vi "Start.vi"(8 "error in (no error)":errorcluster, 11 "Motor-Maxon in":refnum<class "Motor-Maxon.lvclass">) -> (0 "error out":errorcluster, 3 "Motor-Maxon out":refnum<class "Motor-Maxon.lvclass">)   [LabVIEW 2013, in "PowderDeposition.lvlib" / "Motor-Maxon.lvclass"]
uses:
  Motor-Maxon.lvclass
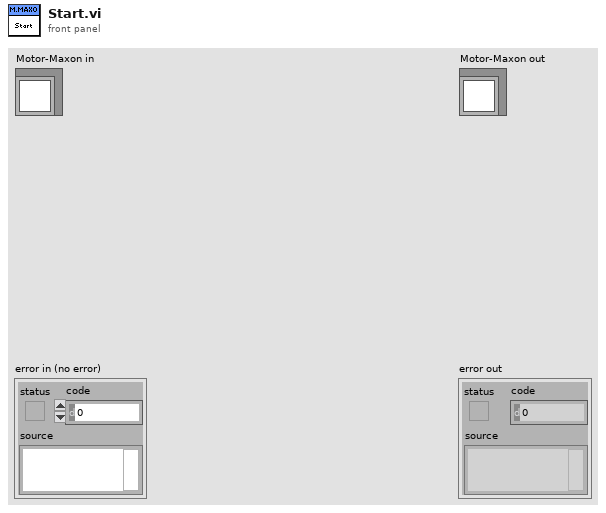
[diagram p1: front panel]
types:
  T1 = cluster{"profileAcceleration":u32, "profileDeceleration":u32}
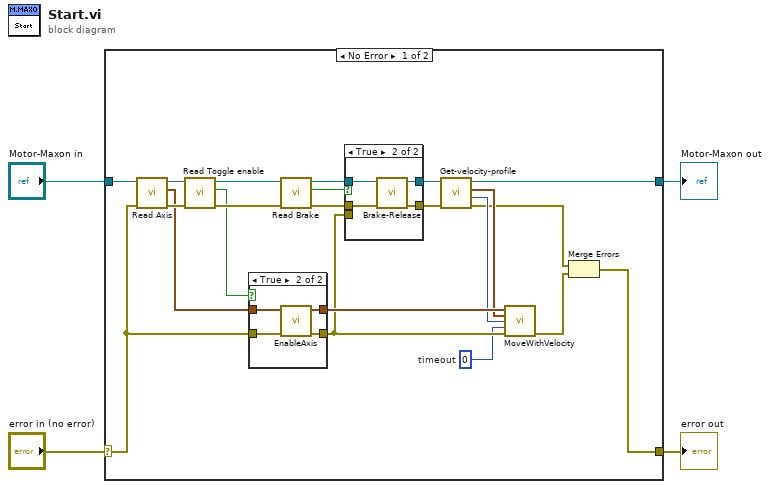
[diagram p0: block diagram]
diagram:
  n1 = case shown="No Error" "error in (no error)" {
    selector: "error in (no error)" -> [w9 w40]
    tunnel: [w26 w40] -> w3
    tunnel: [w7 w39] -> w1
    tunnel: "Motor-Maxon in" -> [w10 w39]
    frame No Error {
      w11 = u32 0  # timeout
      n2 = call-dynamic "Read Axis.vi"("error in (no error)"=w9, "Motor-Maxon in"=w10) -> ("error out"=w24:errorcluster, "Axis"=w23:cluster{"keyHandle":u32, "nodeID":u16}, "Motor-Maxon out"=w25:refnum<class "Motor-Maxon.lvclass">)  [unwired: 7 in]
      n3 = call-dynamic "Read Toggle enable.vi"("error in (no error)"=w24, "Motor-Maxon in"=w25) -> ("error out"=w21:errorcluster, "Toggle enable"=w12:bool, "Motor-Maxon out"=w22:refnum<class "Motor-Maxon.lvclass">)  [unwired: 7 in]
      n4 = case shown="True" w12 {
        tunnel: w23 -> [w34 w37]
        tunnel: w9 -> [w33 w38]
        tunnel: [w34 w36] -> w18
        tunnel: [w33 w35] -> w17
        frame False {
        }
        frame True {
          n5 = call <instrlib>:"EnableAxis.vi"("error in (no error)"=w38, "axis in"=w37) -> ("error out"=w35:errorcluster, "axis out"=w36:cluster{"keyHandle":u32, "nodeId":u16})  [unwired: 4 in]
        }
      }
      n6 = call-dynamic "Read Brake.vi"("error in (no error)"=w21, "Motor-Maxon in"=w22) -> ("error out"=w19:errorcluster, "Brake"=w13:bool, "Motor-Maxon out"=w20:refnum<class "Motor-Maxon.lvclass">)  [unwired: 7 in]
      n7 = case shown="True" w13 {
        tunnel: w20 -> [w28 w32]
        tunnel: w19 -> [w27 w31]
        tunnel: [w28 w30] -> w16
        tunnel: [w27 w29] -> w15
        tunnel: w17 -> [_ _]
        frame False {
        }
        frame True {
          n8 = call-dynamic "Brake-Release.vi"("error in (no error)"=w31, "Motor-Maxon in"=w32) -> ("error out"=w29:errorcluster, "Motor-Maxon out"=w30:refnum<class "Motor-Maxon.lvclass">)  [unwired: 8 in]
        }
      }
      n9 = call-dynamic "Get-velocity-profile.vi"("error in (no error)"=w15, "Motor-Maxon in"=w16) -> ("error out"=w6:errorcluster, "Velocity"=w8:i32, "Velocity profile"=w14:T1, "Motor-Maxon out"=w7:refnum<class "Motor-Maxon.lvclass">)  [unwired: 6 in]
      n10 = call <instrlib>:"MoveWithVelocity.vi"("axis in"=w18, "velocity profile"=w14, "targetVelocity"=w8, "timeout"=w11, "error in (no error)"=w17) -> ("error out"=w5:errorcluster)  [unwired: 9 in, 1 out]
      n11 = Merge Errors(w6, w5) -> (w26:errorcluster)
    }
    frame Error {
    }
  }
  "error out" <- w3
  "Motor-Maxon out" <- w1
